vi "Empty_Queues.vi"(6 "Queues":T1, 8 "Status/Errors in":refnum<vi>, 11 "Device in":refnum<vi>) -> (0 "Status/Errors out":refnum<vi>)   [LabVIEW 2010]
uses:
  Controls/Queues.ctl
  Controls/One_Second.ctl
  Controls/GPS_Timestamp.ctl
  Controls/Device_Elements.ctl
  Controls/Get_Set_Device_Options.ctl
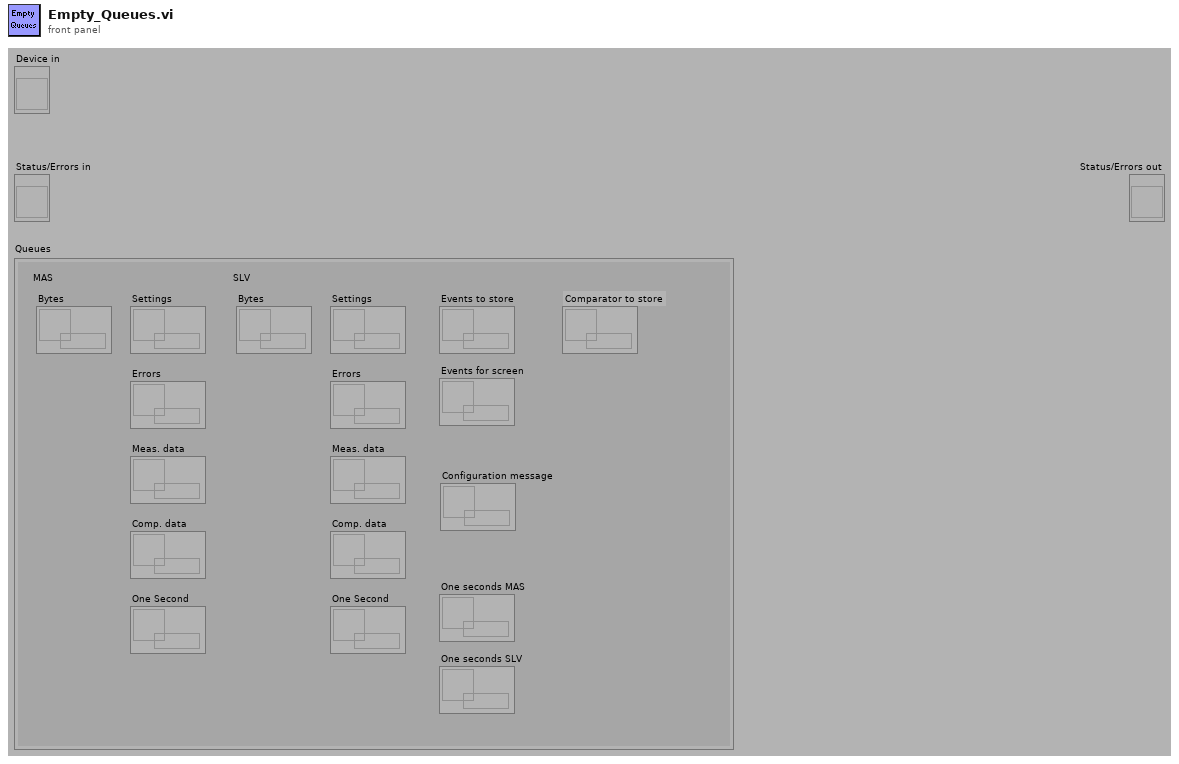
[diagram p1: front panel]
types:
  T1 = typedef "Queues.ctl" = cluster{"MAS":cluster{"Bytes":refnum<queue>, "Settings":refnum<queue>, "Errors":refnum<queue>, "Meas. data":refnum<queue>, "One Second":refnum<queue>, "Comp. data":refnum<queue>}, "SLV":cluster{"Bytes":refnum<queue>, "Settings":refnum<queue>, "Errors":refnum<queue>, "Meas. data":refnum<queue>, "One Second":refnum<queue>, "Comp. data":refnum<queue>}, "Events to store":refnum<queue>, "Events for screen":refnum<queue>, "One seconds MAS":refnum<queue>, "One seconds SLV":refnum<queue>, "Configuration message":refnum<queue>, "Comparator to store":refnum<queue>}
  T2 = typedef "Get_Set_Device_Options.ctl" = enum16{"Get", "Get cluster", "Set"}
  T3 = typedef "Device_Elements.ctl" = enum16{"Default", "Master?", "Connected?", "Status", "Disconnect?", "Handle", "Version number"}
  T4 = typedef "Master.ctl" = enum16{"Master", "Slave", "General"}
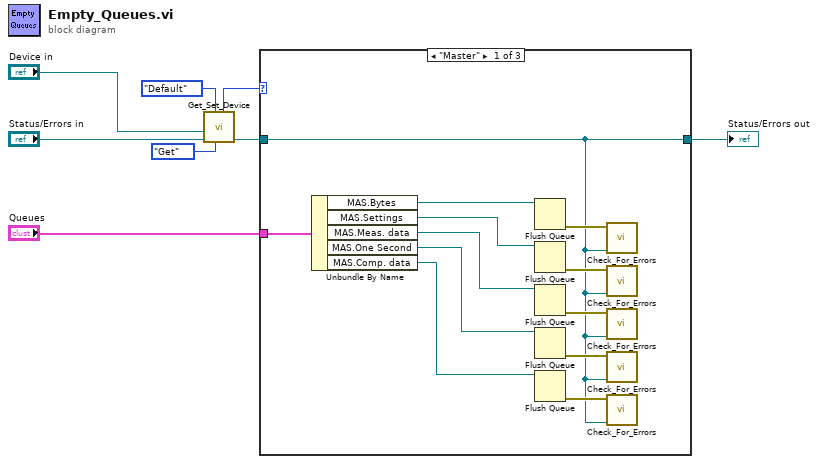
[diagram p0: block diagram]
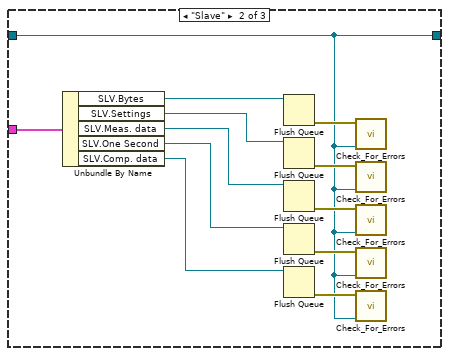
[diagram p2: hidden frame]
diagram:
  n1 = call "Get_Set_Device.vi"("Get/Set"=Get_Set_Device_Options."Get", "Element"=Device_Elements."Default", "Status/Errors in"="Status/Errors in", "Device in"="Device in") -> ("Status/Errors out"=w2:refnum<vi>, "Master?"=w6:T4)  [unwired: 1 in, 5 out]
  n2 = case shown="\"Master\"" w6 {
    tunnel: "Queues" -> [w20 w32 _]
    tunnel: [w10 w22 w33] -> w3
    tunnel: w2 -> [w10 w22 w33]
    frame "Master" {
      n3 = Unbundle By Name(w20) -> ("MAS.Bytes"=w19:refnum<queue>, "MAS.Settings"=w18:refnum<queue>, "MAS.Meas. data"=w17:refnum<queue>, "MAS.One Second"=w16:refnum<queue>, "MAS.Comp. data"=w9:refnum<queue>)
      n4 = Flush Queue(queue=w19) -> (error out=w15:errorcluster)  [unwired: 1 in, 2 out]
      n5 = Flush Queue(queue=w18) -> (error out=w14:errorcluster)  [unwired: 1 in, 2 out]
      n6 = Flush Queue(queue=w17) -> (error out=w13:errorcluster)  [unwired: 1 in, 2 out]
      n7 = Flush Queue(queue=w16) -> (error out=w12:errorcluster)  [unwired: 1 in, 2 out]
      n8 = Flush Queue(queue=w9) -> (error out=w11:errorcluster)  [unwired: 1 in, 2 out]
      n9 = call "Check_For_Errors.vi"("Status/Errors in"=w10, "error in"=w15) -> ()  [unwired: 10 out]
      n10 = call "Check_For_Errors.vi"("Status/Errors in"=w10, "error in"=w14) -> ()  [unwired: 10 out]
      n11 = call "Check_For_Errors.vi"("Status/Errors in"=w10, "error in"=w13) -> ()  [unwired: 10 out]
      n12 = call "Check_For_Errors.vi"("Status/Errors in"=w10, "error in"=w12) -> ()  [unwired: 10 out]
      n13 = call "Check_For_Errors.vi"("Status/Errors in"=w10, "error in"=w11) -> ()  [unwired: 10 out]
    }
    frame "Slave" {
      n14 = Unbundle By Name(w32) -> ("SLV.Bytes"=w31:refnum<queue>, "SLV.Settings"=w30:refnum<queue>, "SLV.Meas. data"=w29:refnum<queue>, "SLV.One Second"=w28:refnum<queue>, "SLV.Comp. data"=w21:refnum<queue>)
      n15 = Flush Queue(queue=w31) -> (error out=w27:errorcluster)  [unwired: 1 in, 2 out]
      n16 = Flush Queue(queue=w30) -> (error out=w26:errorcluster)  [unwired: 1 in, 2 out]
      n17 = Flush Queue(queue=w29) -> (error out=w25:errorcluster)  [unwired: 1 in, 2 out]
      n18 = Flush Queue(queue=w28) -> (error out=w24:errorcluster)  [unwired: 1 in, 2 out]
      n19 = Flush Queue(queue=w21) -> (error out=w23:errorcluster)  [unwired: 1 in, 2 out]
      n20 = call "Check_For_Errors.vi"("Status/Errors in"=w22, "error in"=w27) -> ()  [unwired: 10 out]
      n21 = call "Check_For_Errors.vi"("Status/Errors in"=w22, "error in"=w26) -> ()  [unwired: 10 out]
      n22 = call "Check_For_Errors.vi"("Status/Errors in"=w22, "error in"=w25) -> ()  [unwired: 10 out]
      n23 = call "Check_For_Errors.vi"("Status/Errors in"=w22, "error in"=w24) -> ()  [unwired: 10 out]
      n24 = call "Check_For_Errors.vi"("Status/Errors in"=w22, "error in"=w23) -> ()  [unwired: 10 out]
    }
    frame Default {
    }
  }
  "Status/Errors out" <- w3
